vi "6594 Reference Clock Config.vi"(6 "port number":u8, 8 "error in":errorcluster, 9 "reference clock index":u8, 10 "ref clk frequency":u64, 11 "fpga interface in":refnum<k20>) -> (0 "error out":errorcluster, 3 "fpga interface out":refnum<k20>)   [LabVIEW 2023, in "Aurora64b66b Utilities Host.lvlib"]
uses:
  Aurora64b66b Utilities Host.lvlib
  Program Files/NI/LVAddons/flexrioiia/1/instr.lib/FlexRIO/API/Host/v1/NI FlexRIO API v1.lvlib
  Program Files/NI/LVAddons/flexrioiia/1/instr.lib/FlexRIO/API/Host/v1/NI FlexRIO/API/Get Property Reference - Fpga Small.vi
  <resource>/objmgr/niflexrioapiClock.rc
  <vilib>/ErrorRing/Error Ring.xnode
  <vilib>/Utility/error.llb/Error Cluster From Error Code.vi
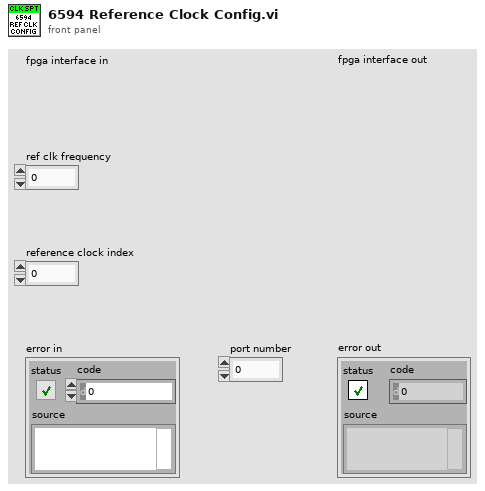
[diagram p1: front panel]
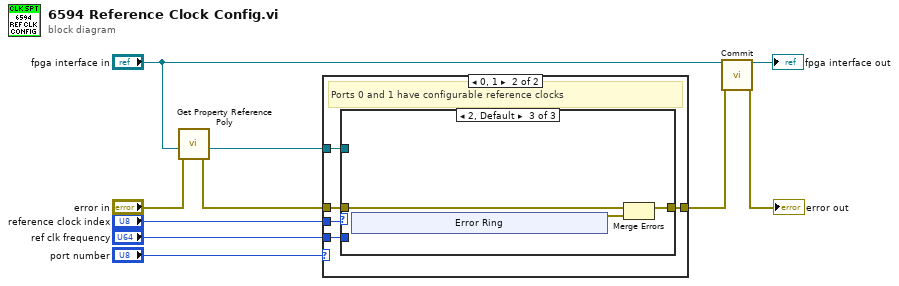
[diagram p0: block diagram]
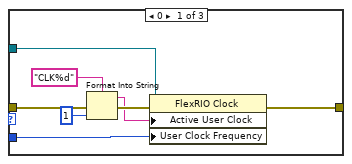
[diagram p3: hidden frame]
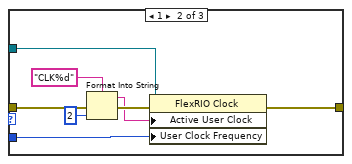
[diagram p4: hidden frame]
diagram:
  n1 = call-poly "Get Property Reference Poly.vi"("error in (no error)"="error in", "fpga interface in"="fpga interface in") -> ("error out"=w6:errorcluster, "property reference"=w5:refnum<k20>)  [unwired: 4 in, 1 out]
  n2 = case shown="0, 1" "port number" {
    tunnel: "reference clock index" -> [_ w16]
    tunnel: w6 -> [w11 w15]
    tunnel: w5 -> [_ w14]
    tunnel: "ref clk frequency" -> [_ w13]
    tunnel: [w11 w12] -> w4
    frame 2, Default {
      # "Port 2 has a fixed 312.5 MHz reference clock. Do nothing"
    }
    frame 0, 1 {
      # "Ports 0 and 1 have configurable reference clocks"
      n3 = case shown="2, Default" w16 {
        tunnel: w15 -> [w21 w29 w35]
        tunnel: [w17 w25 w33] -> w12
        tunnel: w14 -> [w19 w27 _]
        tunnel: w13 -> [w18 w26 _]
        frame 0 {
          n4 = Format Into String(format string="CLK%d" ("Active User Clock"), error in=w21, u8 1 ("input 1")) -> (resulting string=w23:string, error out=w24:errorcluster)  [unwired: 1 in]
          n5 = property class="FlexRIO Clock"(reference=w19, error in=w24, "Active User Clock"=w23, "User Clock Frequency"=w18) -> (error out=w17:errorcluster)  [unwired: 1 out]
        }
        frame 1 {
          n6 = Format Into String(format string="CLK%d" ("Active User Clock"), error in=w29, u8 2 ("input 1")) -> (resulting string=w31:string, error out=w32:errorcluster)  [unwired: 1 in]
          n7 = property class="FlexRIO Clock"(reference=w27, error in=w32, "Active User Clock"=w31, "User Clock Frequency"=w26) -> (error out=w25:errorcluster)  [unwired: 1 out]
        }
        frame 2, Default {
          n8 = xnode "Error Ring"() -> ("error out"=w34:errorcluster)
          n9 = Merge Errors(w35, w34) -> (w33:errorcluster)
        }
      }
    }
  }
  n10 = call "Commit.vi"("fpga interface in"="fpga interface in", "error in"=w4) -> ("fpga interface out"=→"fpga interface out":refnum<k20>, "error out"=→"error out":errorcluster)  [unwired: 12 in]
